vi "Prueba2_GrethelCruz.vi"() -> ()   [LabVIEW 2013]
panel:
  out "MuchoCalor":bool
  out "TemperaturaMayor":dbl
  out "Contador":dbl
  out "TempPromedio":dbl
  out "Thermometer":i32(slide) scale=0.0..60.0
  # "Si tiene que generar la temperatura de todo un dia en intervalos de 2 horas,\nal final del dia debera presentar la temperatura promedio de la temperaturas mayores \na 35 grados y contarlas.\n\nAl final de dia presentar la temperatura mayor.\nCuando la temperatura exceda los 40 grados debera de encender un led.\nEl programa puede detenerse si hay una temperatura arriba de los 55 grados."
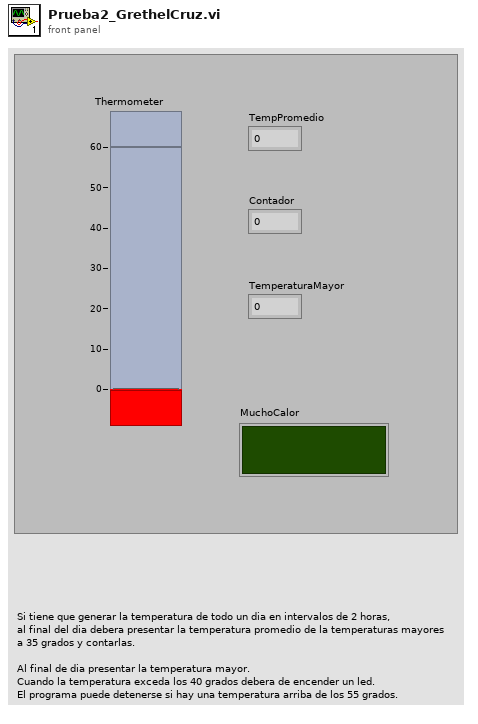
[diagram p1: front panel]
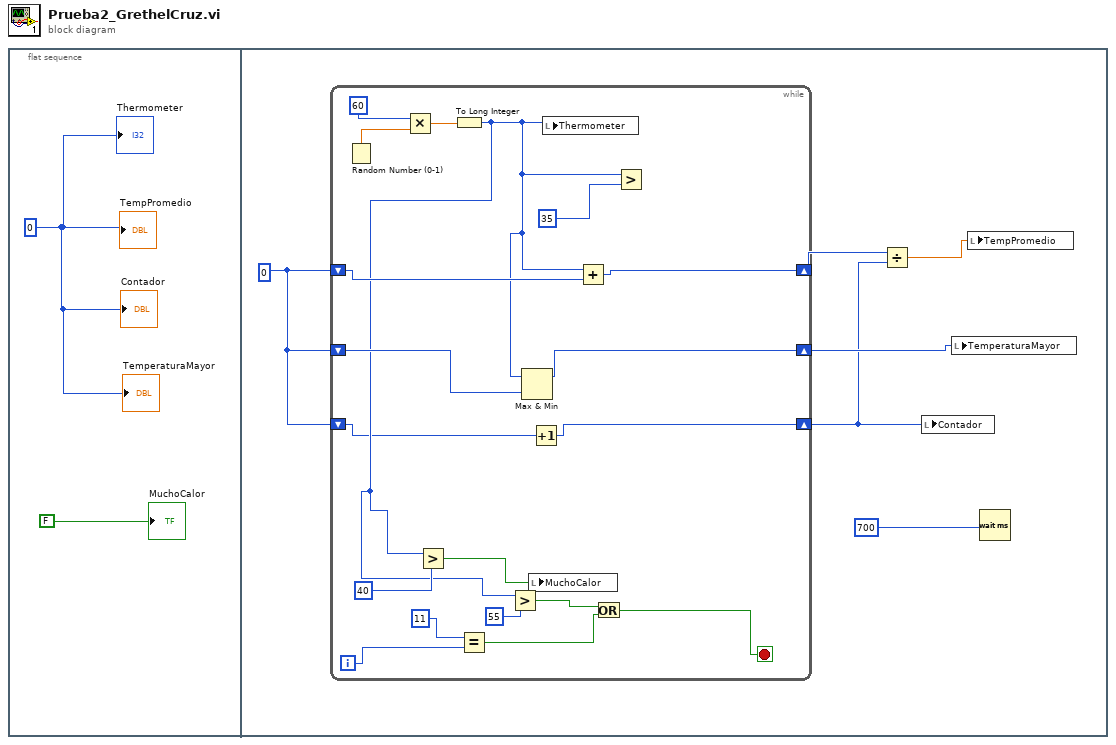
[diagram p0: block diagram]
diagram:
  n1 = flat-sequence {
    frame #0 {
      w2 = 0
      "Thermometer" <- w2
      "TempPromedio" <- w2
      "Contador" <- w2
      "TemperaturaMayor" <- w2
      "MuchoCalor" <- FALSE
    }
    frame #1 {
      w5 = 0
      n2 = while {
        shift-right: [w20] -> w7
        shift-left: w5 -> [w19]
        shift-right: [w18] -> w6
        shift-left: w5 -> [w17]
        shift-right: [w9] -> w4
        shift-left: w5 -> [w10]
        i -> [w16]
        stop <- w13 stop-if-true
        n3 = Random Number (0-1)() -> (number: 0 to 1=w26:dbl)
        n4 = Multiply(x=60, y=w26) -> (x*y=w25:dbl)
        n5 = To Long Integer(number=w25) -> (32bit integer=w14:i32)
        n6 = Greater?(x=w14, y=40) -> (0:w21:bool)
        n7 = Equal?(x=11, y=w16) -> (x = y?=w11:bool)
        n8 = Greater?(x=w14, y=55) -> (0:w12:bool)
        n9 = Max & Min(x=w14, y=w17) -> (max(x,y)=w18:i32)  [unwired: 1 out]
        n10 = local write "MuchoCalor"(w21) -> ()
        n11 = Increment(x=w10) -> (x+1=w9:i32)
        n12 = local write "Thermometer"(w14) -> ()
        n13 = Add(x=w14, y=w19) -> (x+y=w20:i32)
        n14 = Or(x=w12, y=w11) -> (x .or. y?=w13:bool)
        n15 = Greater?(x=w14, y=35) -> ()  [unwired: 1 out]
      }
      n16 = Divide(x=w7, y=w4) -> (x/y=w8:dbl)
      n17 = local write "Contador"(w4) -> ()
      n18 = local write "TemperaturaMayor"(w6) -> ()
      n19 = local write "TempPromedio"(w8) -> ()
      n20 = Wait (ms)(milliseconds to wait=700) -> ()  [unwired: 1 out]
    }
  }
